vi "Test Sector Overlay.vi"() -> ()   [LabVIEW 2013]
uses:
  Test Compiliation/Test Sector Cluster.ctl
panel:
  in  "All":bool
  out "Array":cluster{"X":i32, "Y":i32}[](array[cluster])
  out "size(s)":i32
  in  "Sector":u8
  in  "[Test Sectors]":T1[](array[typedef])
  out "Image":T2(plugin-control)
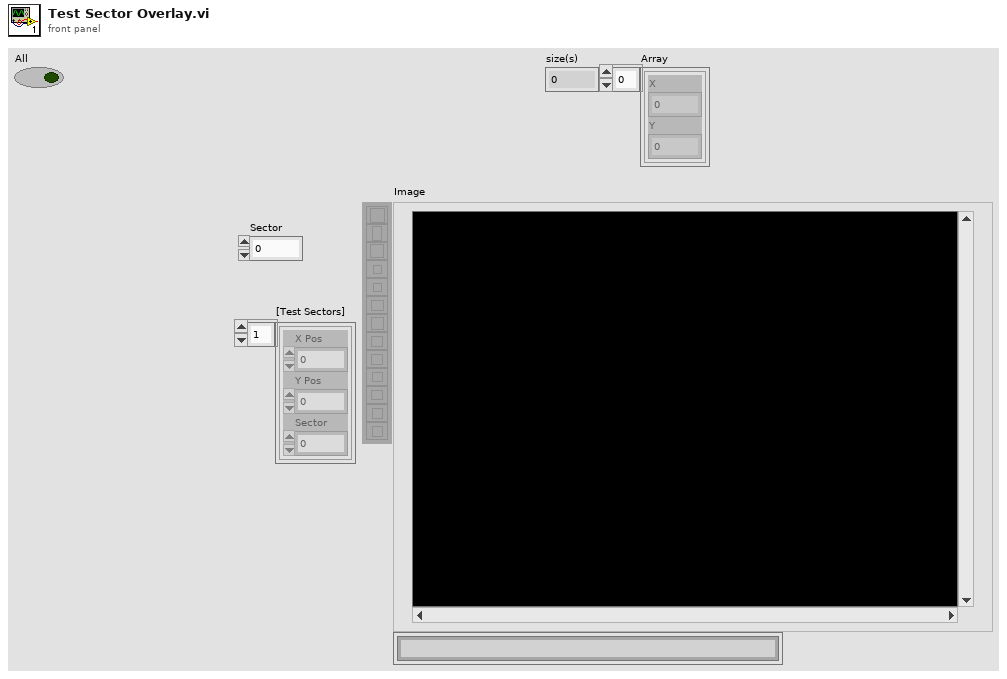
[diagram p1: front panel]
types:
  T1 = typedef "Test Sector Cluster.ctl" = cluster{"X Pos":u16, "Y Pos":u16, "Sector":u8}
  T2 = typedef "IMAQ Image.ctl" = refnum<image>
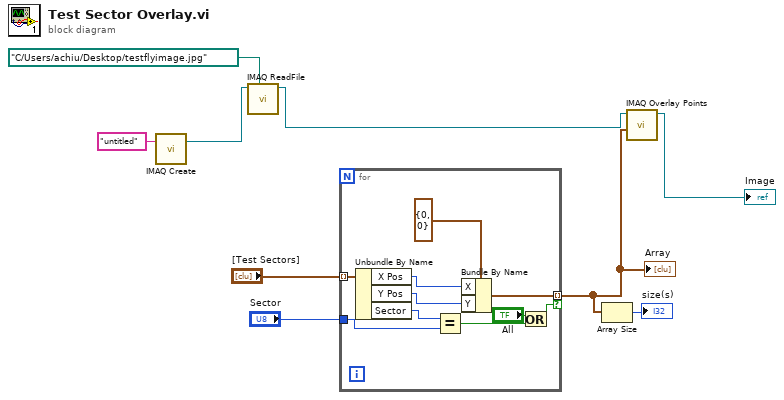
[diagram p0: block diagram]
diagram:
  n1 = call "IMAQ Create"("Image Name"="untitled") -> ("New Image"=w8:T2)  [unwired: 4 in, 1 out]
  n2 = call "IMAQ ReadFile"("File Path"=path "C:/Users/achiu/Desktop/testflyimage.jpg", "Image"=w8) -> ("Image Out"=w6:T2)  [unwired: 5 in, 4 out]
  n3 = for {
    tunnel: "[Test Sectors]" -> [w18] mode=indexing
    tunnel: [w15] -> w2 mode=indexing if=w11
    tunnel: "Sector" -> [w13]
    n4 = Unbundle By Name(w18) -> ("X Pos"=w17:u16, "Y Pos"=w16:u16, "Sector"=w14:u8)
    n5 = Equal?(x=w14, y=w13) -> (x = y?=w12:bool)
    n6 = Bundle By Name(cluster=cluster{"X":i32, "Y":i32} {"X"=0, "Y"=0} ("Point Coordinates"), "X"=w17, "Y"=w16) -> (w15:cluster{"X":i32, "Y":i32})
    n7 = Or(x="All", y=w12) -> (x .or. y?=w11:bool)
  }
  "Array" <- w2
  n8 = Array Size(array=w2) -> (size(s)=→"size(s)":i32)
  n9 = call "IMAQ Overlay Points"("Array of Points"=w2, "Image"=w6) -> ("Image Out"=→"Image":T2)  [unwired: 8 in, 1 out]
